vi "RunProtocolCompletely.vi"(10 "protocol name":string) -> ()   [LabVIEW 2018]
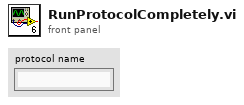
[diagram p1: front panel]
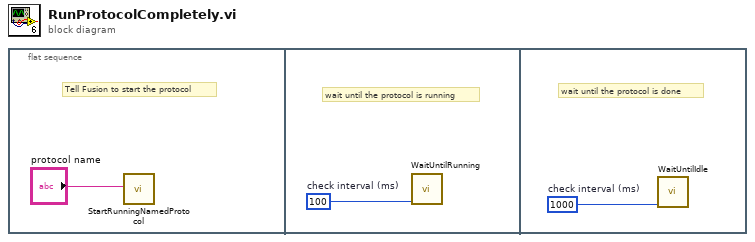
[diagram p0: block diagram]
diagram:
  n1 = flat-sequence {
    frame #0 {
      # "Tell Fusion to start the protocol"
      n2 = call "StartRunningNamedProtocol.vi"("protocol name"="protocol name") -> ()  [unwired: 11 in]
    }
    frame #1 {
      w2 = 100  # check interval (ms)
      # "wait until the protocol is running"
      n3 = call "WaitUntilRunning.vi"("check interval (ms)"=w2) -> ()  [unwired: 11 in]
    }
    frame #2 {
      w3 = 1000  # check interval (ms)
      # "wait until the protocol is done"
      n4 = call "WaitUntilIdle.vi"("check interval (ms)"=w3) -> ()  [unwired: 11 in]
    }
  }
